vi "Plots.vi"() -> ()   [LabVIEW 2019]
uses:
  <vilib>/Utility/file.llb/Write Delimited Spreadsheet (string).vi
  <vilib>/Utility/file.llb/Write Delimited Spreadsheet (DBL).vi
panel:
  out "error out":errorcluster
  in  "stop":bool
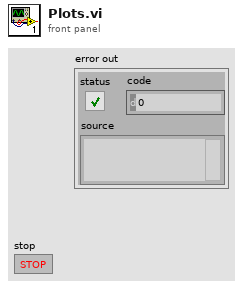
[diagram p1: front panel]
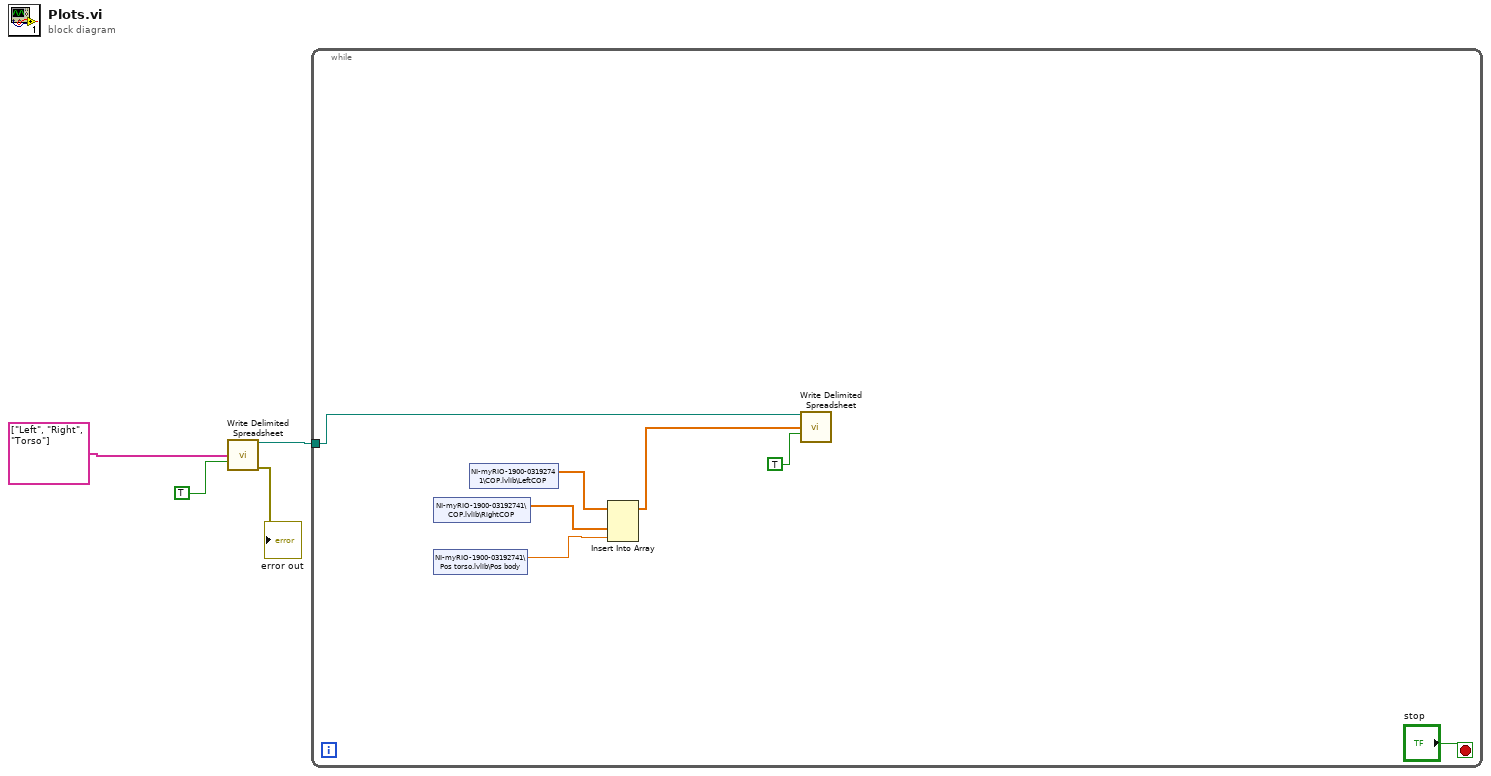
[diagram p0: block diagram]
diagram:
  n1 = call-poly <vilib>:"Write Delimited Spreadsheet.vi"("1D data"=string[] ["Left", "Right", "Torso"], "append to file? (new file:F)"=TRUE) -> ("new file path (Not A Path if cancelled)"=w2:path, "error out"=→"error out":errorcluster)  [unwired: 12 in]
  n2 = while {
    tunnel: w2 -> [w11]
    stop <- "stop" stop-if-true
    n3 = shared-variable "NI-myRIO-1900-03192741\\COP.lvlib\\RightCOP"() -> (w9:dbl[])  [unwired: 1 in, 1 out]
    n4 = shared-variable "NI-myRIO-1900-03192741\\Pos torso.lvlib\\Pos body"() -> (w5:dbl)  [unwired: 1 in, 1 out]
    n5 = shared-variable "NI-myRIO-1900-03192741\\COP.lvlib\\LeftCOP"() -> (w10:dbl[])  [unwired: 1 in, 1 out]
    n6 = Insert Into Array(array=w10, new element #1=w9, new element #2=w5) -> (w8:dbl[])  [unwired: 1 in]
    n7 = call-poly <vilib>:"Write Delimited Spreadsheet.vi"("file path (dialog if empty)"=w11, "1D data"=w8, "append to file? (new file:F)"=TRUE) -> ()  [unwired: 11 in, 2 out]
  }
